vi "Rohde & Schwarz VNA Calibrate.vi"(7 "Rohde & Schwarz VNA":T5, 8 "error in (no error)":errorcluster, 10 "Parameters to Measure":T1[](array[typedef]) {"Channel" min=1 max=99 step=1; "Parameter"."Stimulus Port" min=1 step=1; "Parameter"."Response Port" min=1 step=1}, 11 "VISA Resource Name":refnum<visa-resource-name>) -> (0 "error out":errorcluster {"code" format="%.0x"}, 3 "dup VISA Resource Name":refnum<visa-resource-name>)   [LabVIEW 2011]
uses:
  TypeDefs/Rohde & Schwarz VNA Instrument Info.ctl
  tests/S Parameter/TypeDefs/SP Parameter to Measure.ctl
  tests/S Parameter/TypeDefs/SP Parameter.ctl
  tests/S Parameter/TypeDefs/SP Calibration State.ctl
  tests/S Parameter/TypeDefs/SP Measurement Format.ctl
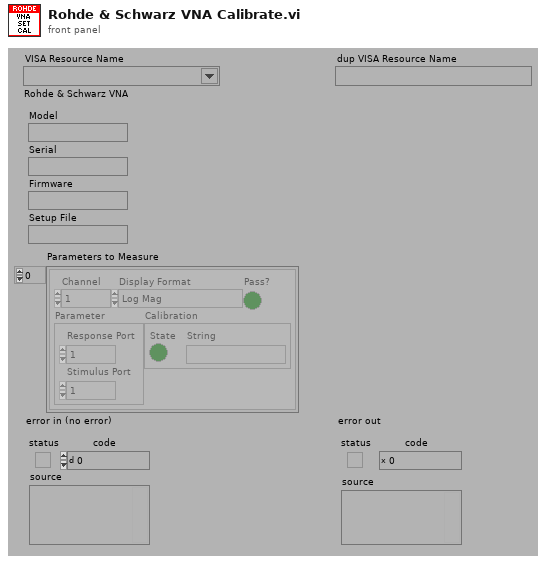
[diagram p1: front panel]
types:
  T1 = typedef "SP Parameter to Measure.ctl" = cluster{"Channel":i8, "Parameter":T2, "Calibration":T3, "Display Format":T4, "Pass?":bool}
  T2 = typedef "SP Parameter.ctl" = cluster{"Stimulus Port":i8, "Response Port":i8}
  T3 = typedef "SP Calibration State.ctl" = cluster{"State":bool, "String":string}
  T4 = typedef "SP Measurement Format.ctl" = enum32{"Log Mag", "Phase", "Delay", "Smith (R+jX)", "Polar (Re/Im)", "Linear Mag", "SWR", "Real", "Imaginary", "Smith (Lin/Phase)", "Smith (Log/Phase)", "Smith (Real/Imag)", "Smith (G+jB)", "Polar (Lin/Phase)", "Polar (Log/Phase)", "Expanded Phase", "Positive Phase", "Inverted Smith", "Unwrapped Phase", "Power Out", "Power In", "Linear Mag/Phase", "Log Mag/Phase", "Real/Imaginary"}
  T5 = typedef "Rohde & Schwarz VNA Instrument Info.ctl" = cluster{"Model":string, "Serial":string, "Firmware":string, "Setup File":string}
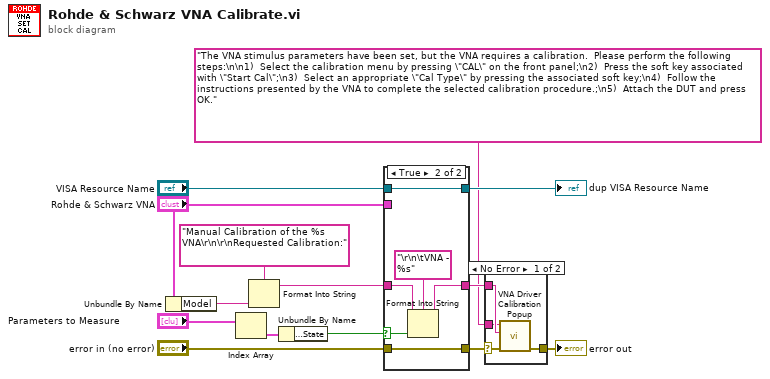
[diagram p0: block diagram]
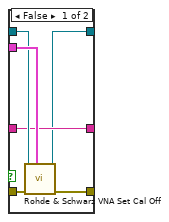
[diagram p2: hidden frame]
diagram:
  n1 = Unbundle By Name("Rohde & Schwarz VNA") -> ("Model"=w6:string)
  n2 = Index Array(array="Parameters to Measure") -> (element=w3:T1)  [unwired: 1 in]
  n3 = Format Into String(format string="Manual Calibration of the %s VNA\r\n\r\nRequested Calibration:", w6) -> (resulting string=w12:string)  [unwired: 2 in, 1 out]
  n4 = Unbundle By Name(w3) -> ("Calibration.State"=w5:bool)
  n5 = case shown="True" w5 {
    selector: w5 -> [_ w21]
    tunnel: w12 -> [w16 w24]
    tunnel: [w16 w26] -> w2
    tunnel: "VISA Resource Name" -> [w19 w23]
    tunnel: "Rohde & Schwarz VNA" -> [w20 _]
    tunnel: "error in (no error)" -> [w18 w25]
    tunnel: [w17 w25] -> w9
    tunnel: [w15 w23] -> w7
    frame False {
      n6 = call "Rohde & Schwarz VNA Set Cal Off.vi"("Rohde & Schwarz VNA"=w20, "error in (no error)"=w18, "VISA Resource Name"=w19) -> ("error out"=w17:errorcluster, "dup VISA Resource Name"=w15:refnum<visa-resource-name>)  [unwired: 7 out]
    }
    frame True {
      n7 = Format Into String(format string="\r\n\tVNA - %s", initial string=w24, w21) -> (resulting string=w26:string)  [unwired: 1 in, 1 out]
    }
  }
  "dup VISA Resource Name" <- w7
  n8 = case shown="No Error" w9 {
    selector: w9 -> [w30 w31]
    tunnel: [w29 w31] -> w14
    tunnel: w2 -> [w28 _]
    tunnel: "The VNA stimulus parameters have been set, but the VNA requires a calibration.  Please perform the following steps:\n\n1)  Select the calibration menu by pressing \"CAL\" on the front panel;\n2)  Press the soft key associated with \"Start Cal\";\n3)  Select an appropriate \"Cal Type\" by pressing the associated soft key;\n4)  Follow the instructions presented by the VNA to complete the selected calibration procedure.;\n5)  Attach the DUT and press OK." -> [w27 _]
    frame No Error {
      n9 = call "VNA Driver Calibration Popup.vi"("error in (no error)"=w30, "RequestedCal"=w28, "Message (\"\")"=w27) -> ("error out"=w29:errorcluster)  [unwired: 8 out]
    }
    frame Error {
    }
  }
  "error out" <- w14
